vi "Read User Events.vi"(8 "error in (no error)":errorcluster, 11 "UI Base in":refnum<class "UI Base.lvclass">) -> (0 "error out":errorcluster, 2 "User Events":cluster{"Stop":refnum<user-event>}, 3 "UI Base out":refnum<class "UI Base.lvclass">)   [LabVIEW 2023, in "UI Base.lvlib" / "UI Base.lvclass"]
uses:
  UI Base.lvclass
  UI Base.lvclass/UI Base.ctl
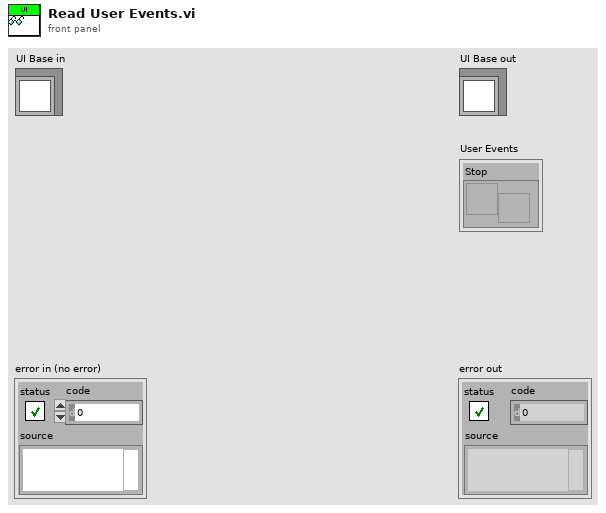
[diagram p1: front panel]
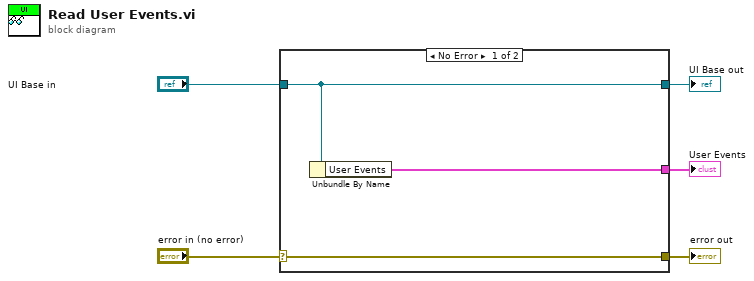
[diagram p0: block diagram]
diagram:
  n1 = case shown="No Error" "error in (no error)" {
    selector: "error in (no error)" -> [w8 w9]
    tunnel: [w8 w9] -> w4
    tunnel: [w7 w10] -> w2
    tunnel: "UI Base in" -> [w7 w10]
    tunnel: [w6 _] -> w1
    frame No Error {
      n2 = Unbundle By Name(w7) -> ("User Events"=w6:cluster{"Stop":refnum<user-event>})
    }
    frame Error {
    }
  }
  "error out" <- w4
  "UI Base out" <- w2
  "User Events" <- w1
